vi "Pulse Output.vi"(3 "Boolean In":bool=TRUE, 4 "Time Target (s)":dbl=1.0) -> (5 "Boolean Out":bool=TRUE)   [LabVIEW 2014]
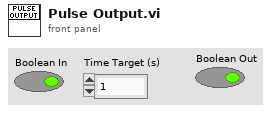
[diagram p1: front panel]
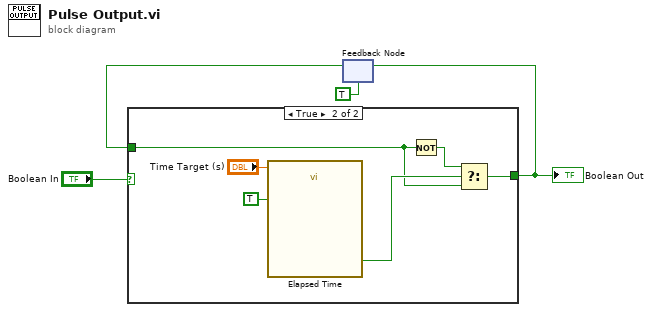
[diagram p0: block diagram]
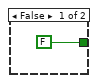
[diagram p2: hidden frame]
diagram:
  n1 = feedback #1(TRUE) -> (w2:bool)
  n2 = case shown="True" "Boolean In" {
    tunnel: [FALSE w7] -> w3
    tunnel: w2 -> [_ w8]
    frame False {
    }
    frame True {
      n3 = call "Elapsed Time"("Time Target (s)"="Time Target (s)", "Auto Reset"=TRUE) -> ("Time has Elapsed"=w10:bool)  [unwired: 10 in, 7 out]
      n4 = Not(x=w8) -> (.not. x?=w9:bool)
      n5 = Select(t=w9, s=w10, f=w8) -> (s? t:f=w7:bool)
    }
  }
  "Boolean Out" <- w3
  n6 = feedback-in #1(w3) -> ()
